vi "x502_out.vi"() -> ()   [LabVIEW 2018]
panel:
  in  "Серийный номер":string
  in  "Channel 2 Signal Params":T1(array[cluster])=[{"Freq"=100.0, "Amp"=2.0, "Phase"=0.0, "Offset"=0.0}]
  in  "Channel 1 Signal Params":T1(array[cluster])=[{"Freq"=1000.0, "Amp"=0.7, "Phase"=0.0, "Offset"=0.0}, {"Freq"=500.0, "Amp"=0.5, "Phase"=0.0, "Offset"=0.0}]
  in  "stop":bool
  in  "Out":bool
  # "По нажатию кнопки OUT происходит установка генерации сигнала в соответствии с заданными параметрами.\nСигнал может быть изменен налету, путем изменения параметров и при повторном нажатии OUT"
  # "Генерируемый сигнал для каждого канала задается как сумма синусоидальных сигналов, для каждого из которых задается частота (Гц), амплитуда (В), начальная фаза (Градусы) и смещение постоянной составляющей (В). Массив сигналов может быть расширен на произвольное число элементов. Если в массиве 0 элементов, то будет выведен сигнал нулевого уровня."
  # "По нажатию STOP (или ошибке вывода) происходит останов генерации и завершение работы с модулем"
  # "По умолчанию программа устранавливает связь с первым найденным E502, подключенным по USB. Если модулей больше одного, то можно ввести серийный номер для явного указания модуля, с которым программа будет работать"
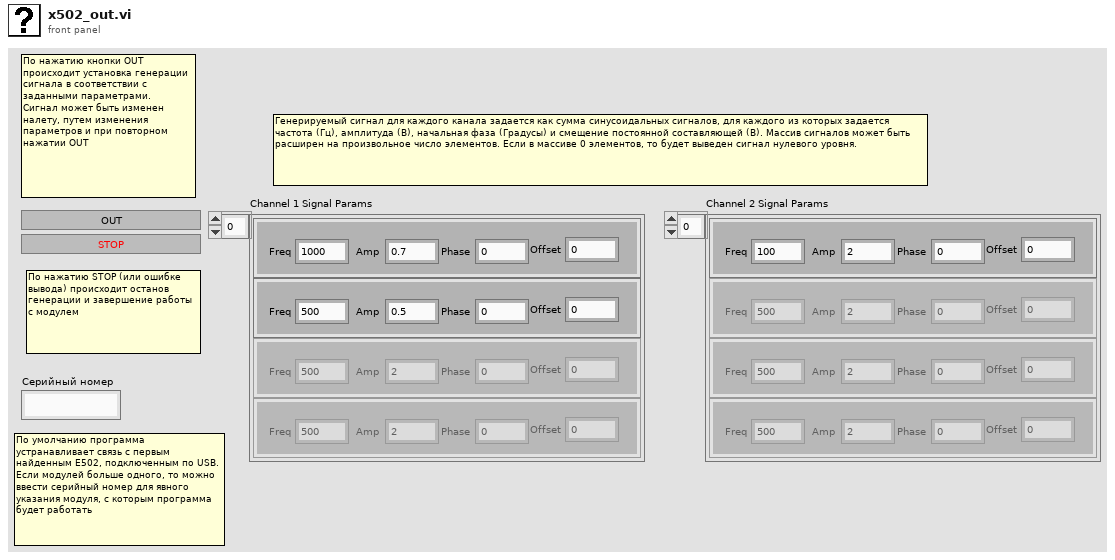
[diagram p1: front panel]
types:
  T1 = cluster{"Freq":dbl, "Amp":dbl, "Phase":dbl, "Offset":dbl}[]
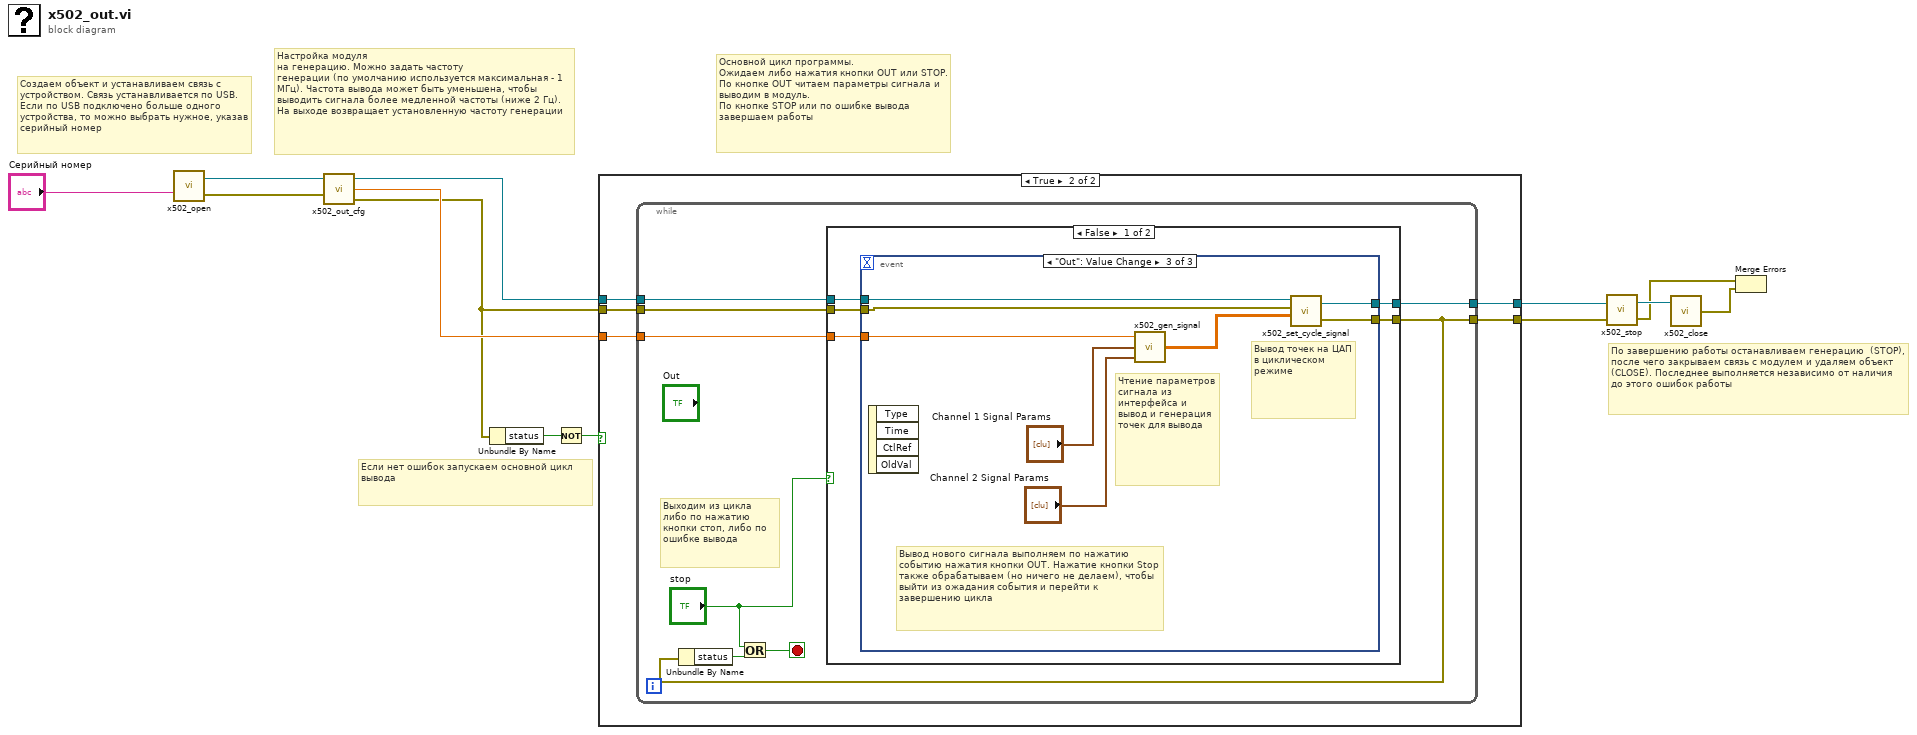
[diagram p0: block diagram]
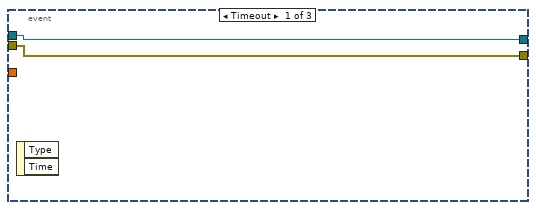
[diagram p3: hidden frame]
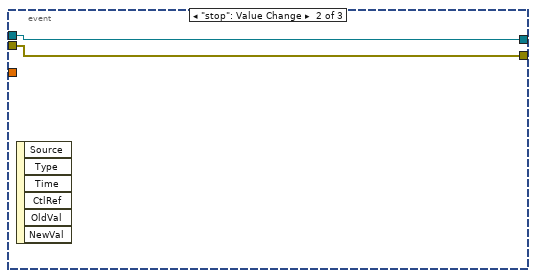
[diagram p4: hidden frame]
diagram:
  # "По завершению работы останавливаем генерацию  (STOP), после чего закрываем связь с модулем и удаляем объект (CLOSE). Последнее выполняется независимо от наличия  до этого ошибок работы"
  # "Основной цикл программы.\nОжидаем либо нажатия кнопки OUT или STOP. По кнопке OUT читаем параметры сигнала и выводим в модуль.\nПо кнопке STOP или по ошибке вывода завершаем работы"
  # "Если нет ошибок запускаем основной цикл вывода"
  # "Настройка модуля\nна генерацию. Можно задать частоту\nгенерации (по умолчанию используется максимальная - 1 МГц). Частота вывода может быть уменьшена, чтобы выводить сигнала более медленной частоты (ниже 2 Гц). На выходе возвращает установленную частоту генерации"
  # "Создаем объект и устанавливаем связь с устройством. Связь устанавливается по USB. Если по USB подключено больше одного устройства, то можно выбрать нужное, указав серийный номер"
  n1 = call "x502_open.vi"("serial"="Серийный номер") -> ("error out"=w11:errorcluster, "x502 out"=w10:refnum<k24>)  [unwired: 1 in]
  n2 = call "x502_out_cfg.vi"("error in (no error)"=w11, "x502 in"=w10) -> ("error out"=w7:errorcluster, "Fout"=w9:dbl, "x502 out"=w8:refnum<k24>)  [unwired: 1 in]
  n3 = Unbundle By Name(w7) -> ("status"=w13:bool)
  n4 = Not(x=w13) -> (.not. x?=w12:bool)
  n5 = case shown="True" w12 {
    tunnel: w9 -> [_ w20]
    tunnel: w8 -> [w15 w19]
    tunnel: w7 -> [w14 w18]
    tunnel: [w15 w17] -> w6
    tunnel: [w14 w16] -> w4
    frame False {
    }
    frame True {
      n6 = while {
        tunnel: w20 -> [w25]
        tunnel: w19 -> [w24]
        tunnel: w18 -> [w23]
        tunnel: [w22] -> w17
        tunnel: [w21] -> w16
        stop <- w27 stop-if-true
        # "Выходим из цикла либо по нажатию кнопки стоп, либо по ошибке вывода"
        n7 = case shown="False" "stop" {
          tunnel: w25 -> [w33 _]
          tunnel: w24 -> [w32 w47]
          tunnel: w23 -> [w31 w46]
          tunnel: [w30 w47] -> w22
          tunnel: [w29 w46] -> w21
          frame False {
            n8 = event shown="[2] \"Out\": Value Change" {
              selector: _ -> [_ _ _]
              dyn-events: _ -> [_ _ _]
              timeout: _ -> [_ _ _]
              tunnel: w33 -> [_ _ w42]
              tunnel: w32 -> [w35 w37 w41]
              tunnel: w31 -> [w34 w36 w40]
              tunnel: [w35 w37 w39] -> w30
              tunnel: [w34 w36 w38] -> w29
              event Timeout {
                n9 = event-data() -> ()  [unwired: 1 in, 2 out]
              }
              event "stop": Value Change {
                n10 = event-data() -> ()  [unwired: 1 in, 6 out]
              }
              event "Out": Value Change {
                # "Вывод точек на ЦАП в циклическом режиме"
                # "Чтение параметров сигнала из интерфейса и вывод и генерация точек для вывода"
                # "Вывод нового сигнала выполняем по нажатию событию нажатия кнопки OUT. Нажатие кнопки Stop также обрабатываем (но ничего не делаем), чтобы выйти из ожадания события и перейти к завершению цикла"
                n11 = event-data() -> ()  [unwired: 1 in, 4 out]
                n12 = call "x502_gen_signal.vi"("Channel 2 Signal Params"="Channel 2 Signal Params", "Channel 1 Signal Params"="Channel 1 Signal Params", "Gen Freq"=w42) -> ("Generated Points"=w43:dbl[][])
                n13 = call "x502_set_cycle_signal.vi"("DAC Signals"=w43, "error in (no error)"=w40, "x502 in"=w41) -> ("error out"=w38:errorcluster, "x502 out"=w39:refnum<k24>)  [unwired: 1 in]
              }
            }
          }
          frame True {
          }
        }
        n14 = Unbundle By Name(w21) -> ("status"=w28:bool)
        n15 = Or(x="stop", y=w28) -> (x .or. y?=w27:bool)
      }
    }
  }
  n16 = call "x502_stop.vi"("error in (no error)"=w4, "x502 in"=w6) -> ("error out"=w3:errorcluster, "x502 out"=w5:refnum<k24>)
  n17 = call "x502_close.vi"("x502 in"=w5) -> ("error out (no error)"=w2:errorcluster)  [unwired: 1 in]
  n18 = Merge Errors(w3, w2) -> ()  [unwired: 1 out]
